vi "DO_Update_Test.vi"() -> ()   [LabVIEW 2020]
uses:
  <vilib>/DAQmx/write.llb/DAQmx Write (Digital U32 1Chan 1Samp).vi
  <vilib>/DAQmx/create/channels.llb/DAQmx Create Channel (DO-Digital Output).vi
  <vilib>/DAQmx/miscellaneous.llb/DAQmx Fill In Error Info.vi
panel:
  in  "Stop":bool
  in  "data":u32=123456 format="%.0x"
  out "error out":errorcluster
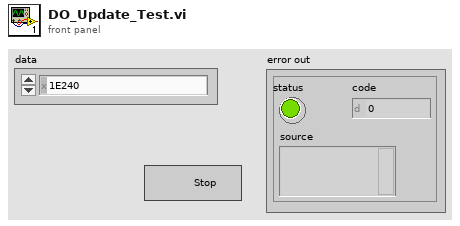
[diagram p1: front panel]
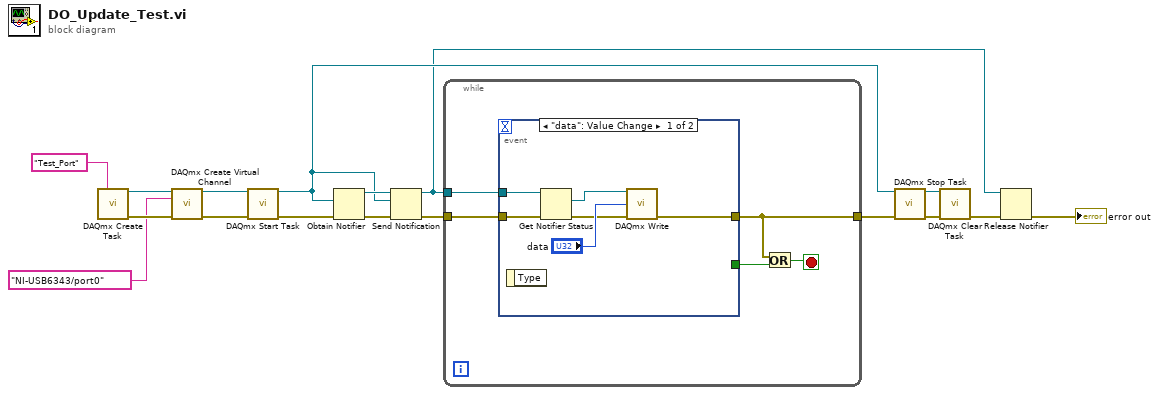
[diagram p0: block diagram]
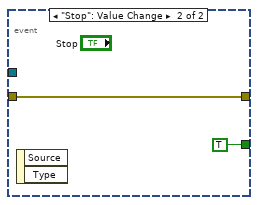
[diagram p2: hidden frame]
diagram:
  n1 = call <vilib>:"DAQmx Create Task.vi"("new task name"="Test_Port") -> ("task out"=w15:refnum<k21>, "error out"=w17:errorcluster)  [unwired: 13 in]
  n2 = call-poly <vilib>:"DAQmx Create Virtual Channel.vi"("task in"=w15, "lines"=tag "NI-USB6343/port0", "error in"=w17) -> ("task out"=w14:refnum<k21>, "error out"=w16:errorcluster)  [unwired: 11 in]
  n3 = call <vilib>:"DAQmx Start Task.vi"("task/channels in"=w14, "error in"=w16) -> ("task out"=w4:refnum<k21>, "error out"=w8:errorcluster)  [unwired: 12 in]
  n4 = Obtain Notifier(notification data type=w4, error in (no error)=w8) -> (notifier out=w5:refnum<notifier>, error out=w7:errorcluster)  [unwired: 2 in, 1 out]
  n5 = Send Notification(notification=w4, notifier=w5, error in (no error)=w7) -> (notifier out=w1:refnum<notifier>, error out=w6:errorcluster)
  n6 = while {
    tunnel: w6 -> [w22]
    tunnel: [w21] -> w11
    tunnel: w1 -> [w18]
    stop <- w19 stop-if-true
    n7 = event shown="[0] \"data\": Value Change" {
      selector: _ -> [_ _]
      dyn-events: _ -> [_ _]
      timeout: _ -> [_ _]
      tunnel: w22 -> [w25 w30]
      tunnel: [w27 w30] -> w21
      tunnel: [_ TRUE] -> w20
      tunnel: w18 -> [w24 _]
      event "data": Value Change {
        n8 = event-data() -> ()  [unwired: 1 in, 1 out]
        n9 = Get Notifier Status(notifier=w24, error in (no error)=w25) -> (current notification=w23:refnum<k21>, error out=w26:errorcluster)  [unwired: 3 out]
        n10 = call-poly <vilib>:"DAQmx Write.vi"("task/channels in"=w23, "data"="data", "error in"=w26) -> ("error out"=w27:errorcluster)  [unwired: 10 in, 2 out]
      }
      event "Stop": Value Change {
        n11 = event-data() -> ()  [unwired: 1 in, 2 out]
      }
    }
    n12 = Or(x=w21, y=w20) -> (x .or. y?=w19:bool)
  }
  n13 = call <vilib>:"DAQmx Stop Task.vi"("task/channels in"=w4, "error in"=w11) -> ("task out"=w9:refnum<k21>, "error out"=w10:errorcluster)  [unwired: 12 in]
  n14 = call <vilib>:"DAQmx Clear Task.vi"("task in"=w9, "error in"=w10) -> ("error out"=w3:errorcluster)  [unwired: 13 in]
  n15 = Release Notifier(notifier=w1, error in (no error)=w3) -> (error out=→"error out":errorcluster)  [unwired: 1 in, 2 out]
